vi "Lock-In Experiment.vi"() -> (0 "K(Indicator)":fxp<+/-,64,32>=1.52587890625e-05, 1 "degree":dbl=0.1952712924057206, 2 "Nominal Freq":fxp<+/-,64,32>=0.494873046875)   [LabVIEW 2012]
uses:
  <vilib>/FPGAPlugInAG/PCI-7831R/niLvFpga_Open_PCI-7831R.vi
  <vilib>/Utility/error.llb/Error Cluster From Error Code.vi
  <vilib>/rvi/errors/niLvFpgaAdjustHostInterfaceError.vi
  <vilib>/FPGAPlugInAG/PCI-7831R/niLvFpga_Run_PCI-7831R.vi
  <vilib>/FPGAPlugInAG/PCI-7831R/niLvFpga_Abort_PCI-7831R.vi
  <vilib>/FPGAPlugInAG/PCI-7831R/niLvFpga_Close_PCI-7831R.vi
  <vilib>/rvi/interface/nirviOpenFPGA/nirviOpenFPGA.xnode
  SB130-XPS/Documents/FPGA-project-apporach-retraction/FPGA Bitfiles/Apporach-Retract_FPGATarget_LIAFPGA3a-PDTest_L-X5ia9B-g4.lvbitx
  LIA_FPGA3a-PD Test.vi
  <vilib>/rvi/interface/nirviReadWriteControl/nirviReadWriteControl.xnode
  <vilib>/rvi/interface/nirviMethod/nirviMethod.xnode
  <vilib>/rvi/interface/nirviCloseFPGA/nirviCloseFPGA.xnode
  NiFpgaLv.dll
panel:
  out "Ref":i32
  out "Sig":i32
  out "Radians":dbl
  out "Cos":dbl(graph)
  out "Sin":dbl(graph)
  out "Phase":dbl
  out "Ze Output":dbl=2.3841857910156248e-12
  out "The Decs":dbl=7.8125e-09
  out "LSB Weight":dbl=0.00030517578125
  in  "K":fxp<+,16,0>=1.52587890625e-05
  in  "nominal freq 2":fxp<+,16,0>=0.494873046875
  out "x*y":dbl=0.015
  in  "stop 2":bool
  out "3rd stages":i32=1
  out "3rd decimation":i32=977
  out "1st decimation":i32=1
  out "2nd decimation":i32=128
  in  "Time Constant [s]":dbl=2.5 min=0.0 step=0.0001 format="%.2f"
  in  "Filter Rolloff":enum16{"20 dB", "40 dB", "60 dB", "80 dB"}(ring)
  out "Actual Sampling Frequency":dbl=200000.0
  in  "input range of 9205":dbl=10.0
  in  "Sampling Frequency":dbl=200000.0 min=1000.0 max=250000.0
  in  "stop":bool
  out "r":dbl(graph)=0.5098420210496609
  out "y":dbl=0.0017376029872894286
  out "x":dbl=0.5098390600609779
  out "f":dbl(graph)=31000.332441180944
  in  "dec2":i16=1
  in  "nominal freq":dbl=30000.0 min=500.0 max=125000.0
  in  "dec1":i16=1000
  in  "stages":i8=1 min=1 max=2
  in  "decimation":i16=1000
  # "Sampling Frequency"
  # "CIC First Decimation"
  # "CIC Second Decimation"
  # "MA Stages"
  # "MA Decimation"
  # "PLL Nominal Frequency"
  # "PLL Frequency Output"
  # "LIA Output"
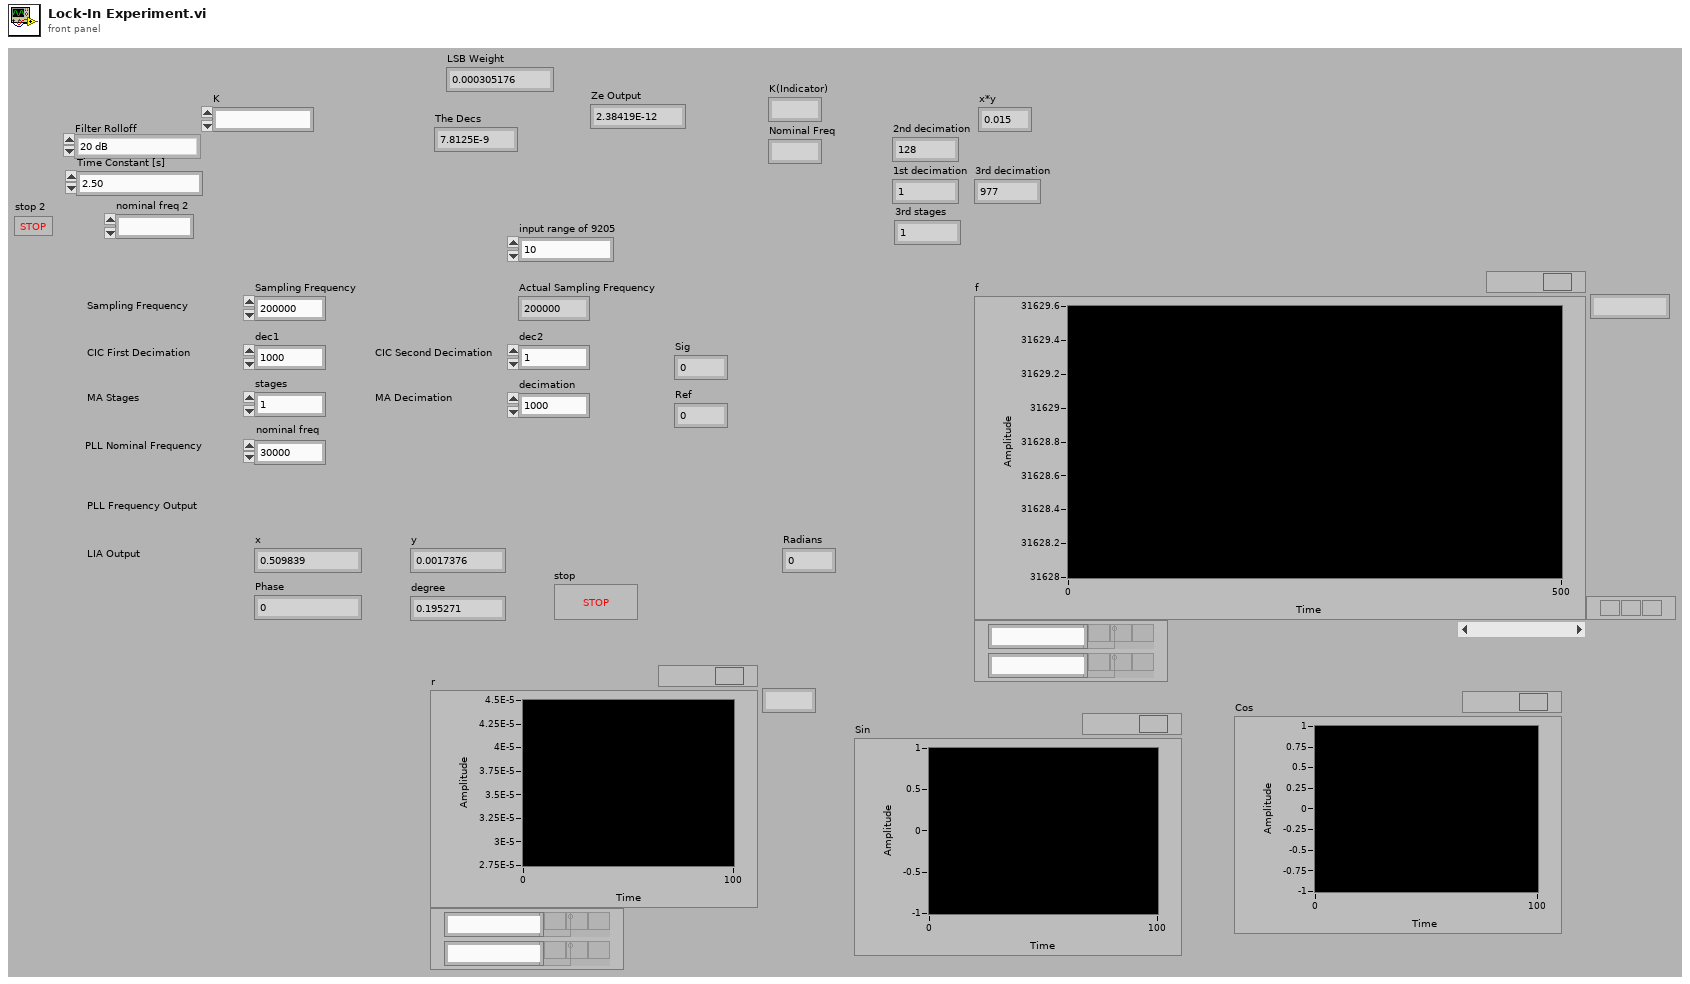
[diagram p1: front panel]
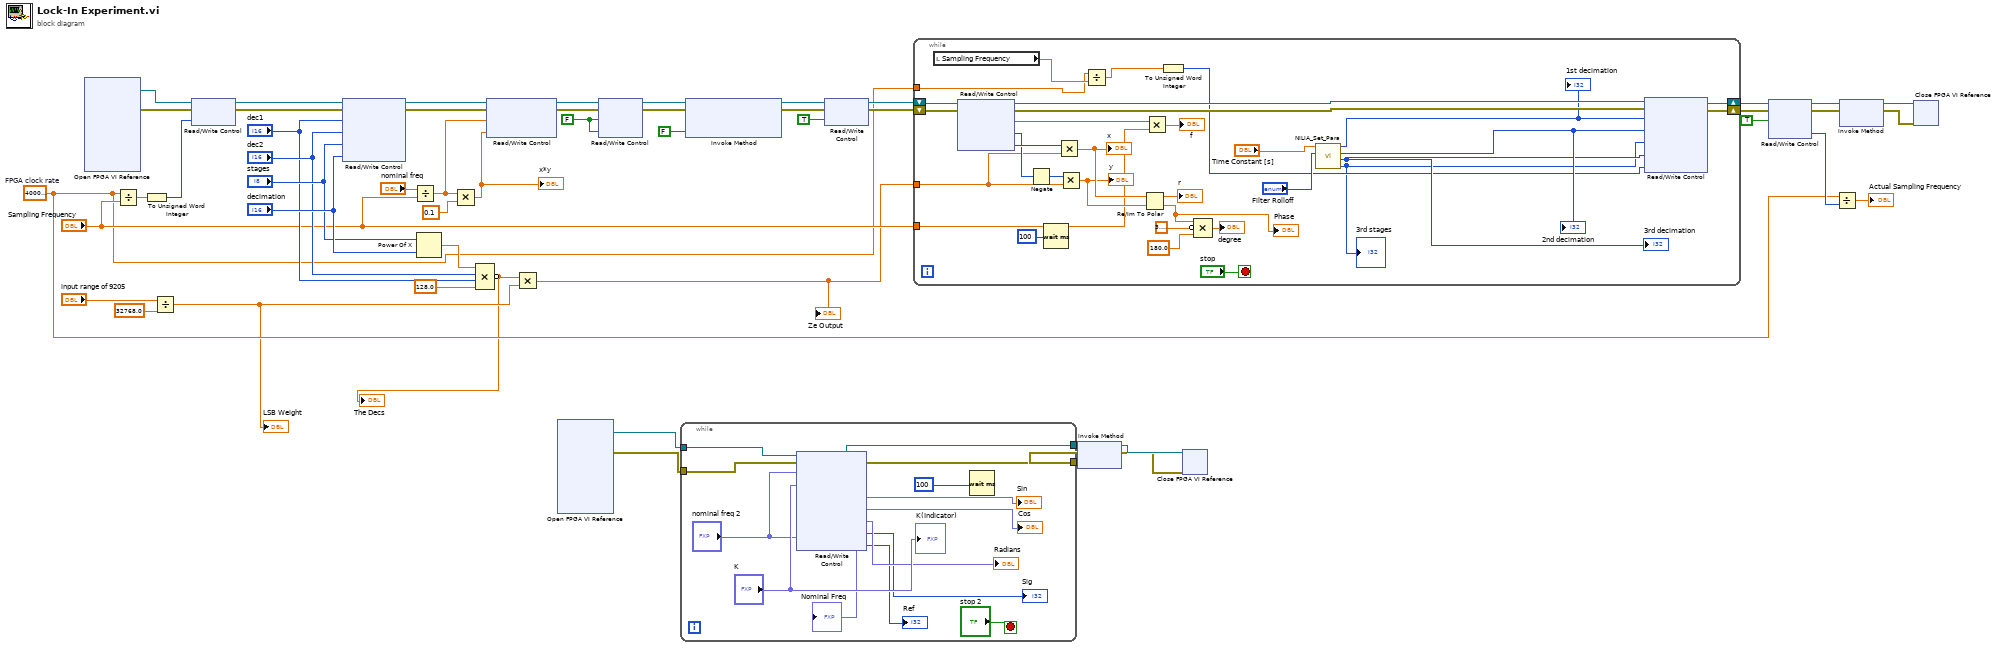
[diagram p0: block diagram]
diagram:
  w11 = 40000000.0  # FPGA clock rate
  w30 = FALSE ("start")
  n1 = xnode "Open FPGA VI Reference"() -> ("FPGA VI Reference Out"=w17:refnum<k20>, "error out"=w16:errorcluster)  [unwired: 2 in]
  n2 = Divide(x=w11, y="Sampling Frequency") -> (x/y=w23:dbl)
  n3 = To Unsigned Word Integer(number=w23) -> (unsigned 16bit integer=w22:u16)
  n4 = Divide(x="input range of 9205", y=32768.0) -> (x/y=w3:dbl)
  "LSB Weight" <- w3
  n5 = xnode "Read/Write Control"("FPGA VI Reference In"=w17, "error in"=w16, "Period"=w22) -> ("FPGA VI Reference Out"=w25:refnum<k20>, "error out"=w24:errorcluster)
  n6 = xnode "Read/Write Control"("FPGA VI Reference In"=w25, "error in"=w24, "dec1"="dec1", "dec2"="dec2", "stages"="stages", "decimation"="decimation") -> ("FPGA VI Reference Out"=w51:refnum<k20>, "error out"=w50:errorcluster)
  n7 = Divide(x="nominal freq", y="Sampling Frequency") -> (x/y=w19:dbl)
  n8 = Power Of X(1:"decimation", 2:"stages") -> (0:w46:dbl)
  n9 = Multiply(x=w19, y=0.1) -> (x*y=w4:dbl)
  "x*y" <- w4
  n10 = Compound Arithmetic op=MULTIPLY(w46, "dec2", "dec1", 128.0) -> (invert w2:dbl)
  "The Decs" <- w2
  n11 = xnode "Read/Write Control"("FPGA VI Reference In"=w51, "error in"=w50, "nominal freq"=w19, "K"=w4) -> ("FPGA VI Reference Out"=w34:refnum<k20>, "error out"=w33:errorcluster)
  n12 = Multiply(x=w2, y=w3) -> (x*y=w1:dbl)
  "Ze Output" <- w1
  n13 = xnode "Open FPGA VI Reference"() -> ("FPGA VI Reference Out"=w10:refnum<k20>, "error out"=w9:errorcluster)  [unwired: 2 in]
  n14 = xnode "Read/Write Control"("FPGA VI Reference In"=w34, "error in"=w33, "start"=w30, "stop"=w30) -> ("FPGA VI Reference Out"=w32:refnum<k20>, "error out"=w31:errorcluster)
  n15 = while {
    tunnel: w10 -> [w63]
    tunnel: w9 -> [w62]
    tunnel: [w61] -> w8
    tunnel: [w60] -> w7
    stop <- "stop 2" stop-if-true
    n16 = xnode "Read/Write Control"("FPGA VI Reference In"=w63, "error in"=w62, "nominal freq"="nominal freq 2", "K"="K") -> ("FPGA VI Reference Out"=w61:refnum<k20>, "error out"=w60:errorcluster, "Sin"=→"Sin":fxp<+/-,14,2>, "Cos"=→"Cos":fxp<+/-,14,2>, "Radians"=→"Radians":fxp<+/-,14,5>, "sig"=→"Sig":i16, "ref"=→"Ref":i16)
    n17 = Wait (ms)(milliseconds to wait=u32 100) -> ()  [unwired: 1 out]
    "K(Indicator)" <- "K"
    "Nominal Freq" <- "nominal freq 2"
  }
  n18 = xnode "Invoke Method"("FPGA VI Reference In"=w32, "error in"=w31, "Wait Until Done (F)"=FALSE) -> ("FPGA VI Reference Out"=w39:refnum<k20>, "error out"=w37:errorcluster)
  n19 = xnode "Read/Write Control"("FPGA VI Reference In"=w39, "error in"=w37, "start"=TRUE) -> ("FPGA VI Reference Out"=w38:refnum<k20>, "error out"=w36:errorcluster)
  n20 = while {
    shift-right: [w77] -> w42
    shift-left: w38 -> [w94]
    shift-right: [w76] -> w41
    shift-left: w36 -> [w93]
    tunnel: w1 -> [w90]
    tunnel: "Sampling Frequency" -> [w80]
    tunnel: w11 -> [w69]
    stop <- "stop" stop-if-true
    n21 = local read "Sampling Frequency"() -> (w70:dbl)
    n22 = xnode "Read/Write Control"("FPGA VI Reference In"=w94, "error in"=w93) -> ("FPGA VI Reference Out"=w77:refnum<k20>, "error out"=w76:errorcluster, "f"=w81:fxp<+/-,32,0>, "channelQ"=w91:i64, "channelI"=w92:i64)
    n23 = Negate(x=w91) -> (-x=w78:i64)
    n24 = Wait (ms)(milliseconds to wait=u32 100) -> ()  [unwired: 1 out]
    n25 = Multiply(x=w92, y=w90) -> (x*y=w89:dbl)
    "x" <- w89
    n26 = Multiply(x=w78, y=w90) -> (x*y=w88:dbl)
    "y" <- w88
    n27 = Divide(x=w69, y=w70) -> (x/y=w68:dbl)
    n28 = Re/Im To Polar(2:w88, 3:w89) -> (0:w65:dbl, 1:→"r":dbl)
    "Phase" <- w65
    n29 = Multiply(x=w81, y=w80) -> (x*y=→"f":dbl)
    n30 = To Unsigned Word Integer(number=w68) -> (unsigned 16bit integer=w67:u16)
    n31 = Compound Arithmetic op=MULTIPLY(w65, invert 3.141592653589793, 180.0 ("value")) -> (→"degree":dbl)
    n32 = call "NILIA_Set_Para.vi"("rolloff"="Filter Rolloff", "TC [sec]"="Time Constant [s]") -> ("3rd stages"=w66:i32, "3rd decimation"=w71:i32, "2nd decimation"=w72:i32, "1st decimation"=w73:i32)  [unwired: 5 in, 1 out]
    "2nd decimation" <- w72
    "1st decimation" <- w73
    "3rd decimation" <- w71
    "3rd stages" <- w66
    n33 = xnode "Read/Write Control"("FPGA VI Reference In"=w77, "error in"=w76, "dec1"=w73, "dec2"=w72, "stages"=w66, "decimation"=w71, "Period"=w67) -> ()  [unwired: 2 out]
  }
  n34 = xnode "Invoke Method"("FPGA VI Reference In"=w8, "error in"=w7) -> ("FPGA VI Reference Out"=w6:refnum<k20>, "error out"=w5:errorcluster)
  n35 = xnode "Close FPGA VI Reference"("FPGA VI Reference In"=w6, "error in"=w5) -> ()  [unwired: 1 out]
  n36 = xnode "Read/Write Control"("FPGA VI Reference In"=w42, "error in"=w41, "stop"=TRUE) -> ("FPGA VI Reference Out"=w29:refnum<k20>, "error out"=w28:errorcluster, "ticks"=w13:u16)
  n37 = Divide(x=w11, y=w13) -> (x/y=→"Actual Sampling Frequency":dbl)
  n38 = xnode "Invoke Method"("FPGA VI Reference In"=w29, "error in"=w28) -> ("FPGA VI Reference Out"=w27:refnum<k20>, "error out"=w26:errorcluster)
  n39 = xnode "Close FPGA VI Reference"("FPGA VI Reference In"=w27, "error in"=w26) -> ()  [unwired: 1 out]
